vi "RBVASS2mk3.vi"() -> ()   [LabVIEW 2021]
uses:
  <vilib>/myRIO/Instrument Drivers/Onboard IO/AI/AI.lvlib
  <vilib>/myRIO/Common/Instrument Driver Framework/Utilities/typedefs/Analog Scaling Constants.ctl
  <vilib>/myRIO/Common/Instrument Driver Framework/Utilities/typedefs/Analog Scaling Constants List.ctl
  <vilib>/myRIO/Common/Instrument Driver Framework/myRIO v1.0/AI/typedefs/AI Channels Enum.ctl
  <vilib>/myRIO/Common/Instrument Driver Framework/myRIO v1.0/AI/typedefs/AI Channels List.ctl
  <vilib>/myRIO/Common/Instrument Driver Framework/Utilities/typedefs/Generic FPGA Reference.ctl
  <vilib>/myRIO/Common/Instrument Driver Framework/Utilities/typedefs/myRIO v1.0 Reference.ctl
  <vilib>/myRIO/Common/Instrument Driver Framework/Utilities/typedefs/Hardware Version Enum.ctl
  <vilib>/myRIO/Common/Instrument Driver Framework/Utilities/typedefs/myRIO Generic Hardware Reference.ctl
  <vilib>/myRIO/Instrument Drivers/Onboard IO/AI/typedefs/AI Reference.ctl
  <vilib>/myRIO/Instrument Drivers/Onboard IO/AI/vis/myRIO AI Open.xnode
  <vilib>/myRIO/Common/Instrument Driver Framework/myRIO v1.0/AI/vis/myRIO v1.1 Open AI.vi
  <vilib>/userDefined/High Color/nirio_resource_hc.ctl
  <vilib>/vision/driver/NI_Vision_Acquisition_Software.lvlib
  <vilib>/vision/NI_Vision_Development_Module.lvlib
  <vilib>/myRIO/Instrument Drivers/Onboard IO/PWM/PWM.lvlib
  <vilib>/vision/driver/IMAQdx.llb/IMAQdx Camera Control Mode.ctl
  <vilib>/vision/driver/IMAQdx.llb/IMAQdx Acquisition Mode.ctl
  <vilib>/vision/driver/IMAQdx.llb/IMAQdx Buffer Number Mode.ctl
  <vilib>/myRIO/Instrument Drivers/Onboard IO/PWM/typedefs/PWM Configuration.ctl
  <vilib>/myRIO/Common/Instrument Driver Framework/myRIO v1.0/PWM/typedefs/PWM Channels Enum.ctl
  <vilib>/myRIO/Instrument Drivers/Onboard IO/PWM/typedefs/PWM Reference.ctl
  <vilib>/myRIO/Instrument Drivers/Onboard IO/PWM/vis/myRIO PWM Open.xnode
  <vilib>/myRIO/Common/Instrument Driver Framework/myRIO v1.0/PWM/vis/myRIO v1.1 Open PWM.vi
  <vilib>/userDefined/High Color/IMAQdx.ctl
  <vilib>/myRIO/Instrument Drivers/Onboard IO/DIO/DIO.lvlib
  Example VI (1)/t_state.ctl
  <vilib>/myRIO/Common/Instrument Driver Framework/myRIO v1.0/DIO/typedefs/DIO Channels Enum.ctl
  <vilib>/myRIO/Common/Instrument Driver Framework/myRIO v1.0/DIO/typedefs/DIO Channels List.ctl
  <vilib>/myRIO/Instrument Drivers/Onboard IO/DIO/typedefs/DIO Reference.ctl
  <vilib>/myRIO/Common/Instrument Driver Framework/myRIO v1.0/DIO/vis/myRIO v1.1 Open DIO.vi
  <vilib>/myRIO/Instrument Drivers/Onboard IO/DIO/vis/myRIO DIO Open.xnode
  Example VI (1)/t_conn.ctl
panel:
  out "circles":i32
  in  "ROI Descriptor":T1 {"Contours"."Type" items=["No Selection", "Point", "Line", "Rectangle", "Oval", "Polygon", "Freehand Region", "Annulus", "Unused2", "Unused3", "Broken Line", "Freehand Line", "Rotated Rectangle"]}
  out "Image 2":T2(plugin-control)
  in  "error in 2":errorcluster
  in  "Settings":T3={"Objects"=0, "Threshold"=128, "Reject Border"=FALSE, "Fill Holes"=FALSE, "Min Object Size"=FALSE, "Min Size"=3, "Max Object Size"=FALSE, "Max Size"=100, "Show Search Area"=FALSE, "Show Center"=TRUE, "Show Bounding Box"=TRUE} {"Objects" items=["Bright Objects", "Dark Objects"]; "Threshold" min=1 max=999999999 step=1; "Max Size" min=1 max=999999999 step=1; "Min Size" min=1 max=999999999 step=1}
  in  "error in":errorcluster
  in  "stop":bool
  out "object":i32
  out "Colour Value":u32
  out "Color Box":u32(colorbox)
  in  "Knob":dbl(knob) scale=0.0..180.0
  out "error out":errorcluster
  out "Slide":dbl(slide) scale=0.0..10.0
  out "Numeric":i32
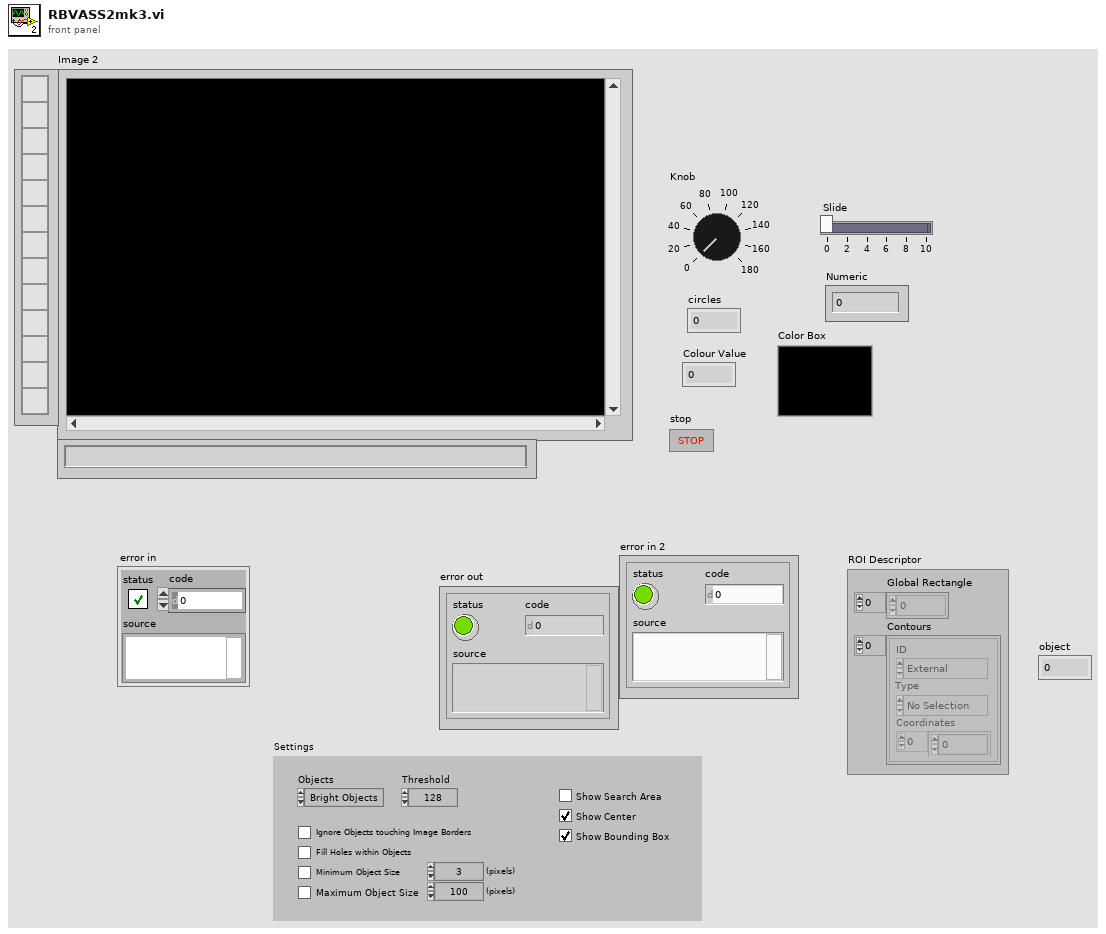
[diagram p1: front panel]
types:
  T1 = cluster{"Global Rectangle":i32[], "Contours":cluster{"ID":enum32{"External", "Internal"}, "Type":u32, "Coordinates":i32[]}[]}
  T2 = typedef "IMAQ Image.ctl" = refnum<image>
  T3 = cluster{"Objects":u16, "Threshold":i32, "Reject Border":bool, "Fill Holes":bool, "Min Object Size":bool, "Min Size":i32, "Max Object Size":bool, "Max Size":i32, "Show Search Area":bool, "Show Center":bool, "Show Bounding Box":bool}
  T4 = typedef "t_conn.ctl" = cluster{"ID":refnum<k5>, "Conn.":bool}
  T5 = typedef "t_state.ctl" = enum16{"Wait for Disconnect", "Stop Listen", "Listen", "Start Listen"}
  T6 = typedef "IMAQdx.ctl" = refnum<k21>
  T7 = typedef "NI_Vision_Acquisition_Software.lvlib/IMAQdx Buffer Number Mode.ctl" = enum32{"Next", "Last", "Buffer Number", "Every", "Last New"}
  T8 = typedef "NI_Vision_Acquisition_Software.lvlib/IMAQdx Acquisition Mode.ctl" = enum32{"One Shot", "Continuous"}
  T9 = typedef "NI_Vision_Acquisition_Software.lvlib/IMAQdx Camera Control Mode.ctl" = enum32{"Controller", "Listener"}
  T10 = typedef "DIO.lvlib/DIO Reference.ctl" = cluster{"myRIO Reference":T11, "DIO Channels List":T15}
  T11 = typedef "myRIO Generic Hardware Reference.ctl" = cluster{"myRIO Model":T12, "myRIO Hardware Reference":T13}
  T12 = typedef "Hardware Version Enum.ctl" = enum16{"Unknown", "myRIO-1900", "myRIO-1950", "roboRIO", "NI ELVIS RIO CM", "ELVIS III"}
  T13 = typedef "myRIO v1.0 Reference.ctl" = cluster{"Generic FPGA Reference":T14, "Allow multiple opens":bool}
  T14 = typedef "Generic FPGA Reference.ctl" = refnum<k20>
  T15 = typedef "DIO Channels List.ctl" = T16[]
  T16 = typedef "DIO Channels Enum.ctl" = enum16{"Not Connected", "C/DIO0", "C/DIO1", "C/DIO2", "C/DIO3", "C/DIO4", "C/DIO5", "C/DIO6", "C/DIO7", "A/DIO0", "A/DIO1", "A/DIO2", "A/DIO3", "A/DIO4", "A/DIO5", "A/DIO6", "A/DIO7", "A/DIO8", "A/DIO9", "A/DIO10", "A/DIO11", "A/DIO12", "A/DIO13", "A/DIO14", "A/DIO15", "A/DIO16", "A/DIO17", "A/DIO18", "A/DIO19", "B/DIO0", "B/DIO1", "B/DIO2", "B/DIO3", "B/DIO4", "B/DIO5", "B/DIO6", "B/DIO7", "B/DIO8", "B/DIO9", "B/DIO10", "B/DIO11", "B/DIO12", "B/DIO13", "B/DIO14", "B/DIO15", "B/DIO16", "B/DIO17", "B/DIO18", "B/DIO19", "LED0", "LED1", "LED2", "LED3", "Button0", "DIO/DIO0", "DIO/DIO1", "DIO/DIO2", "DIO/DIO3", "DIO/DIO4", "DIO/DIO5", "DIO/DIO6", "DIO/DIO7", "DIO/DIO8", "DIO/DIO9", "SPI/CS0", "SPI/CS1", "SPI/CS2", "SPI/CS3", "LED RADIO (Green)", "LED RADIO (Red)", "LED COMM (Green)", "LED COMM (Red)", "LED MODE (Green)", "LED MODE (Red)"}
  T17 = typedef "PWM.lvlib/PWM Reference.ctl" = cluster{"myRIO Reference":T11, "PWM Channels Enum":T18, "PWM Configuration":T19}
  T18 = typedef "PWM Channels Enum.ctl" = enum16{"Not Connected", "C/PWM0", "C/PWM1", "A/PWM0", "A/PWM1", "A/PWM2", "A/PWM3", "A/PWM4", "A/PWM5", "A/PWM6", "A/PWM7", "A/PWM8", "A/PWM9", "A/PWM10", "A/PWM11", "A/PWM12", "A/PWM13", "A/PWM14", "A/PWM15", "A/PWM16", "A/PWM17", "A/PWM18", "A/PWM19", "B/PWM0", "B/PWM1", "B/PWM2", "B/PWM3", "B/PWM4", "B/PWM5", "B/PWM6", "B/PWM7", "B/PWM8", "B/PWM9", "B/PWM10", "B/PWM11", "B/PWM12", "B/PWM13", "B/PWM14", "B/PWM15", "B/PWM16", "B/PWM17", "B/PWM18", "B/PWM19", "PWM/PWM0", "PWM/PWM1", "PWM/PWM2", "PWM/PWM3", "PWM/PWM4", "PWM/PWM5", "PWM/PWM6", "PWM/PWM7", "PWM/PWM8", "PWM/PWM9"}
  T19 = typedef "PWM.lvlib/PWM Configuration.ctl" = cluster{"Frequency":dbl, "Duty Cycle":dbl}
  T20 = typedef "AI.lvlib/AI Reference.ctl" = cluster{"myRIO Reference":T11, "AI Channels List":T21, "AI Scaling Constants List":T23}
  T21 = typedef "AI Channels List.ctl" = T22[]
  T22 = typedef "AI Channels Enum.ctl" = enum16{"Not Connected", "AudioIn/Left", "AudioIn/Right", "C/AI0", "C/AI1", "A/AI0", "A/AI1", "A/AI2", "A/AI3", "A/AI4", "A/AI5", "A/AI6", "A/AI7", "B/AI0", "B/AI1", "B/AI2", "B/AI3", "B/AI4", "B/AI5", "B/AI6", "B/AI7", "AI/AI0", "AI/AI1", "AI/AI2", "AI/AI3", "A/AI0 (DIFF)", "A/AI1 (DIFF)", "A/AI2 (DIFF)", "A/AI3 (DIFF)", "B/AI0 (DIFF)", "B/AI1 (DIFF)", "B/AI2 (DIFF)", "B/AI3 (DIFF)"}
  T23 = typedef "Analog Scaling Constants List.ctl" = T24[]
  T24 = typedef "Analog Scaling Constants.ctl" = cluster{"LSB Weight (Volts)":dbl, "Offset (Volts)":dbl, "Signed?":bool}
  T25 = typedef "Image Type" = u32
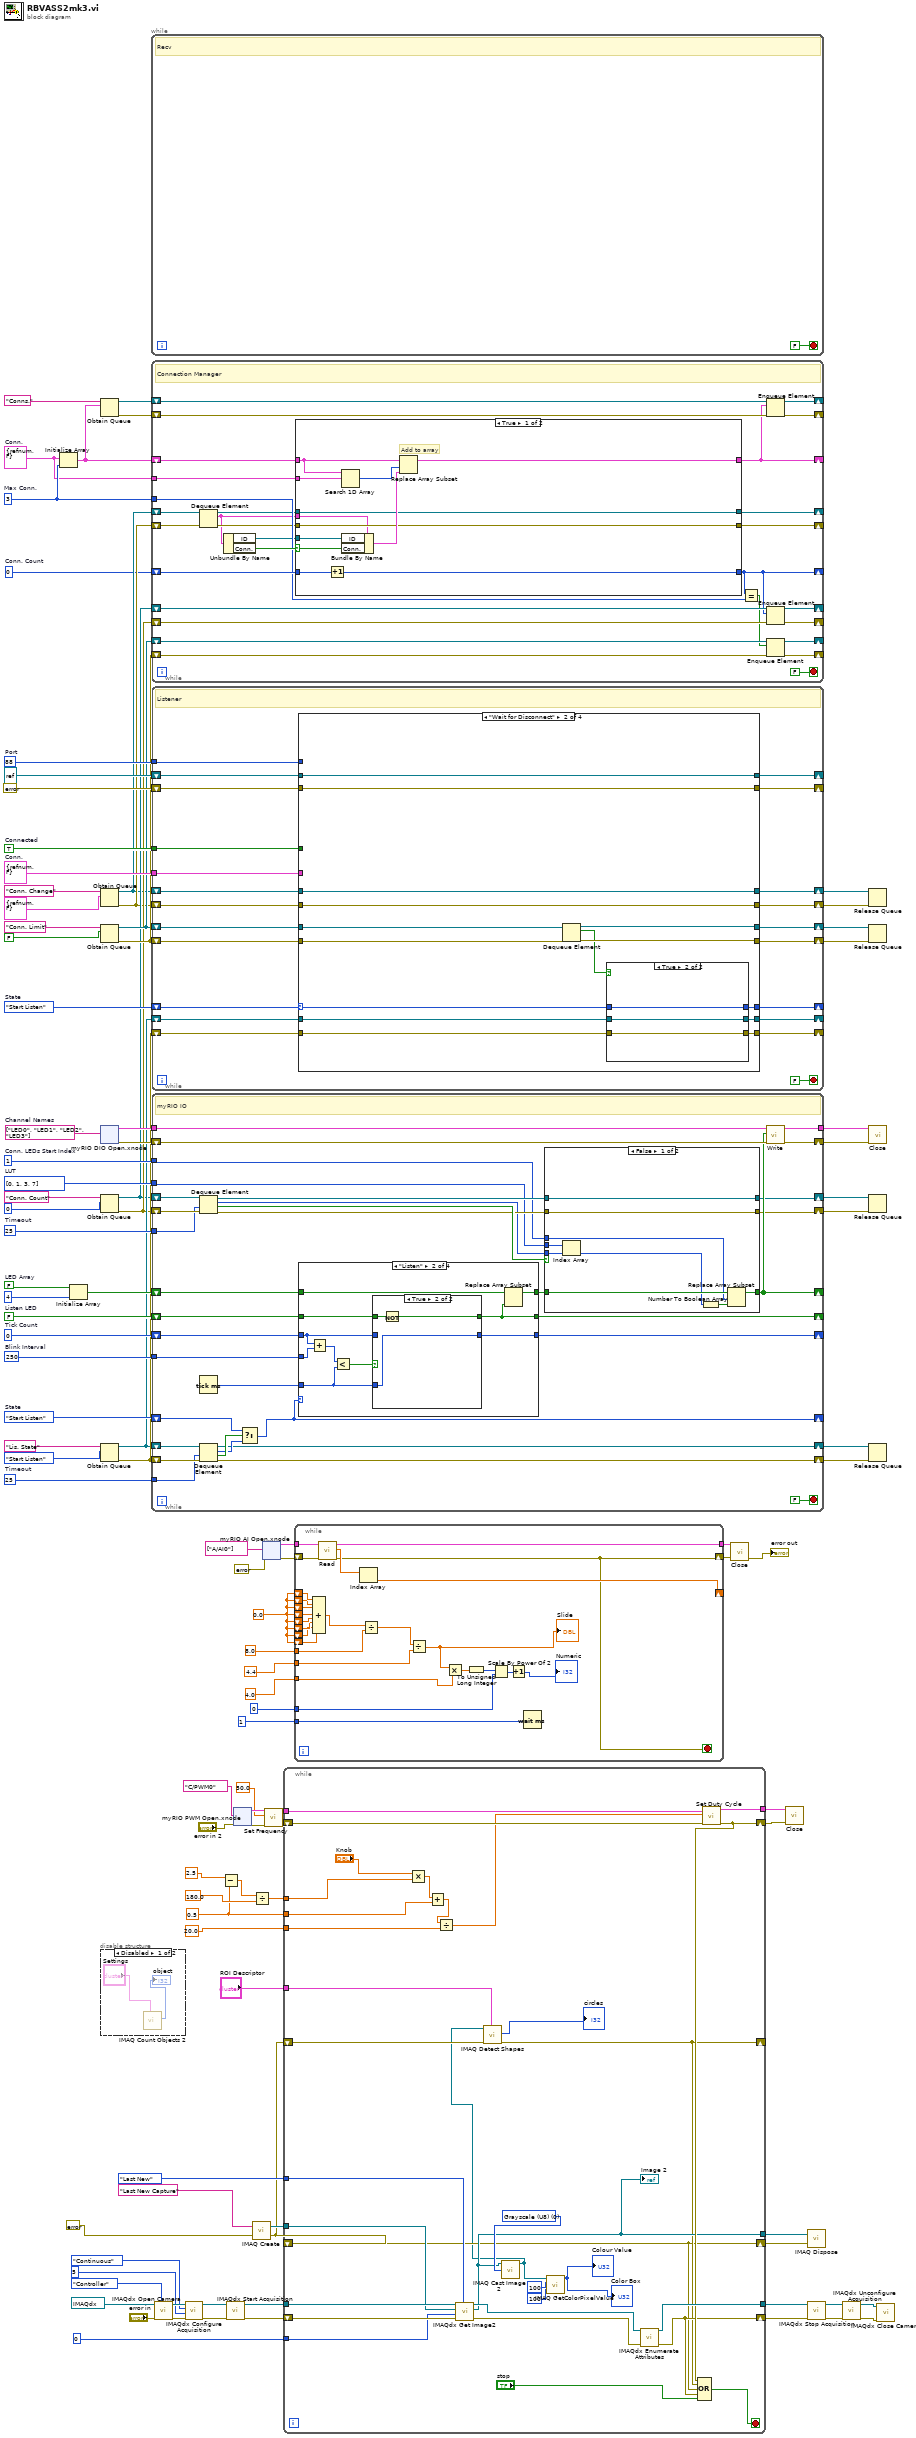
[diagram p0: block diagram]
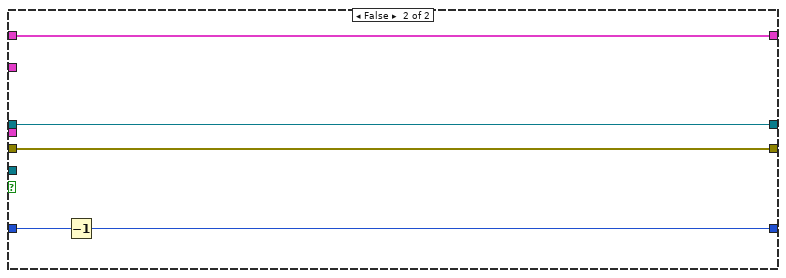
[diagram p2: hidden frame]
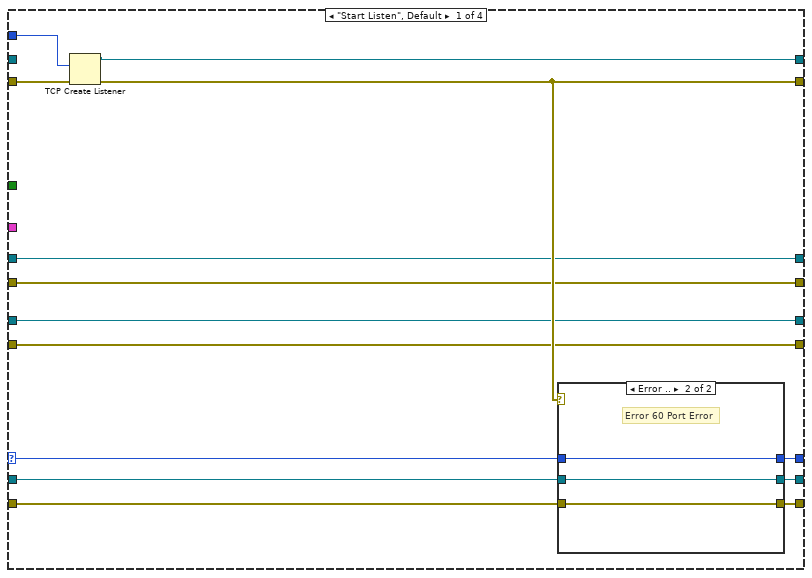
[diagram p3: hidden frame]
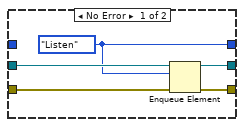
[diagram p4: hidden frame]
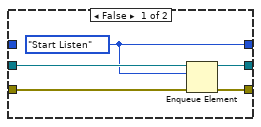
[diagram p5: hidden frame]
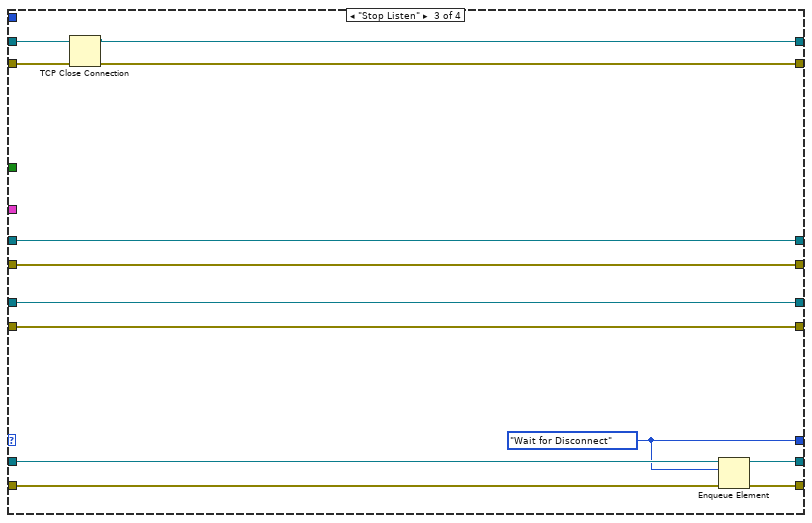
[diagram p6: hidden frame]
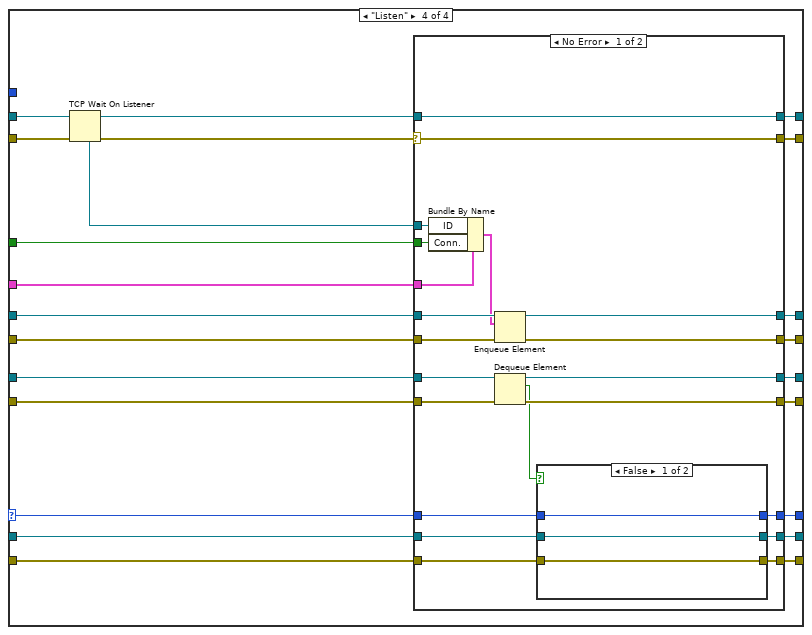
[diagram p7: hidden frame]
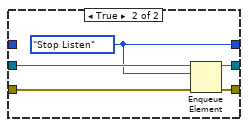
[diagram p8: hidden frame]
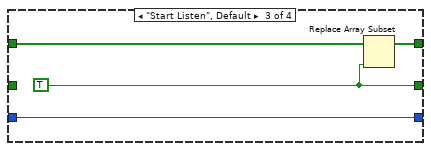
[diagram p13: hidden frame]
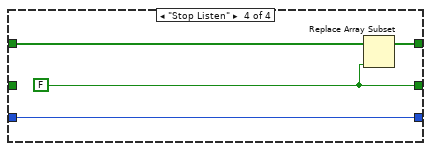
[diagram p14: hidden frame]
diagram:
  w3 = 0  # Conn. Count
  w2 = 3  # Max Conn.
  w1 = T4 {"ID"=refnum, "Conn."=FALSE}  # Conn.
  w18 = TRUE  # Connected
  w24 = u16 88  # Port
  w27 = t_state."Start Listen"  # State
  w19 = T4 {"ID"=refnum, "Conn."=FALSE}  # Conn.
  w32 = 25  # Timeout
  w37 = 25  # Timeout
  w40 = u32 250  # Blink Interval
  w41 = u32 0  # Tick Count
  w42 = t_state."Start Listen"  # State
  w43 = FALSE  # Listen LED
  w44 = i32[] [0, 1, 3, 7]  # LUT
  w45 = 1  # Conn. LEDs Start Index
  w46 = tag[] ["LED0", "LED1", "LED2", "LED3"]  # Channel Names
  w48 = FALSE  # LED Array
  w57 = 0.5
  w101 = 0.0
  n1 = Initialize Array(w1, w2) -> (w4:T4[])
  n2 = Initialize Array(w48, 4 ("dimension size")) -> (w47:bool[])
  n3 = Obtain Queue(name (unnamed)="Conns.", element data type=w4) -> (queue out=w6:refnum<queue>, error out=w7:errorcluster)  [unwired: 3 in, 1 out]
  n4 = Obtain Queue(name (unnamed)="Conn. Change", element data type=T4 {"ID"=refnum, "Conn."=FALSE} ("Conn.")) -> (queue out=w8:refnum<queue>, error out=w9:errorcluster)  [unwired: 3 in, 1 out]
  n5 = Obtain Queue(name (unnamed)="Conn. Limit", element data type=FALSE) -> (queue out=w12:refnum<queue>, error out=w13:errorcluster)  [unwired: 3 in, 1 out]
  n6 = xnode "myRIO DIO Open.xnode"("Channel Names"=w46) -> ("error out"=w53:errorcluster, "DIO Ref Out"=w51:T10)  [unwired: 2 in]
  n7 = Obtain Queue(name (unnamed)="Conn. Count", element data type=0) -> (queue out=w10:refnum<queue>, error out=w11:errorcluster)  [unwired: 3 in, 1 out]
  n8 = Obtain Queue(name (unnamed)="Lis. State", element data type=t_state."Start Listen" ("State")) -> (queue out=w28:refnum<queue>, error out=w29:errorcluster)  [unwired: 3 in, 1 out]
  n9 = disable-structure shown="Disabled" {
    frame Disabled {
      n10 = call "IMAQ Count Objects 2"("Settings"="Settings") -> ("Number of Objects"=→"object":i32)  [unwired: 6 in, 4 out]
    }
    frame Enabled {
    }
  }
  n11 = while {
    stop <- FALSE stop-if-true
    # "Recv"
  }
  n12 = while {
    shift-right: [w135] -> _
    shift-left: w13 -> [w136]
    shift-right: [w133] -> _
    shift-left: w12 -> [w134]
    shift-right: [w131] -> _
    shift-left: w11 -> [w132]
    shift-right: [w129] -> _
    shift-left: w10 -> [w130]
    shift-right: [w113] -> _
    shift-left: w8 -> [w137]
    shift-right: [w115] -> _
    shift-left: w9 -> [w138]
    shift-right: [w125] -> _
    shift-left: w6 -> [w126]
    shift-right: [w127] -> _
    shift-left: w7 -> [w128]
    shift-right: [w111] -> _
    shift-left: w4 -> [w119]
    shift-right: [w122] -> _
    shift-left: w3 -> [w123]
    tunnel: w2 -> [w120]
    tunnel: w1 -> [w118]
    stop <- FALSE stop-if-true
    # "Connection Manager"
    n13 = Dequeue Element(queue=w137, error in (no error)=w138) -> (queue out=w114:refnum<queue>, element=w112:T4, error out=w116:errorcluster)  [unwired: 1 in, 1 out]
    n14 = Unbundle By Name(w112) -> ("ID"=w117:refnum<k5>, "Conn."=w124:bool)
    n15 = case shown="True" w124 {
      selector: w124 -> [w145 _]
      tunnel: w123 -> [w151 w156]
      tunnel: [w150 w155] -> w122
      tunnel: w119 -> [w149 w152]
      tunnel: w118 -> [w146 _]
      tunnel: [w148 w152] -> w111
      tunnel: w117 -> [w144 _]
      tunnel: [w142 w154] -> w115
      tunnel: w116 -> [w142 w154]
      tunnel: w114 -> [w141 w153]
      tunnel: [w141 w153] -> w113
      tunnel: w112 -> [w140 _]
      frame True {
        # "Add to array"
        n16 = Increment(x=w151) -> (x+1=w150:i32)
        n17 = Search 1D Array(1D array=w149, element=w146) -> (index of element=w147:i32)  [unwired: 1 in]
        n18 = Bundle By Name(cluster=w140, "ID"=w144, "Conn."=w145) -> (w143:T4)
        n19 = Replace Array Subset(array=w149, new element=w143, index=w147) -> (w148:T4[])
      }
      frame False {
        n20 = Decrement(x=w156) -> (x-1=w155:i32)
      }
    }
    n21 = Equal?(x=w122, y=w120) -> (x = y?=w121:bool)
    n22 = Enqueue Element(queue=w126, element=w111, error in (no error)=w128) -> (queue out=w125:refnum<queue>, error out=w127:errorcluster)  [unwired: 1 in, 1 out]
    n23 = Enqueue Element(queue=w130, element=w122, error in (no error)=w132) -> (queue out=w129:refnum<queue>, error out=w131:errorcluster)  [unwired: 1 in, 1 out]
    n24 = Enqueue Element(queue=w134, element=w121, error in (no error)=w136) -> (queue out=w133:refnum<queue>, error out=w135:errorcluster)  [unwired: 1 in, 1 out]
  }
  n25 = while {
    shift-right: [w170] -> _
    shift-left: w29 -> [w171]
    shift-right: [w168] -> _
    shift-left: w28 -> [w169]
    shift-right: [w167] -> _
    shift-left: w27 -> [w177]
    shift-right: [w174] -> _
    shift-left: refnum<k5> refnum ("listener ID") -> [w175]
    shift-right: [w173] -> _
    shift-left: errorcluster {"status"=FALSE, "code"=0, "source"=""} ("error constant") -> [w176]
    tunnel: w24 -> [w172]
    shift-right: [w159] -> w14
    shift-left: w8 -> [w160]
    shift-right: [w161] -> w15
    shift-left: w9 -> [w162]
    shift-right: [w163] -> w16
    shift-left: w12 -> [w164]
    shift-right: [w165] -> w17
    shift-left: w13 -> [w166]
    tunnel: w19 -> [w158]
    tunnel: w18 -> [w157]
    stop <- FALSE stop-if-true
    # "Listener"
    n26 = case shown="\"Wait for Disconnect\"" w177 {
      selector: w177 -> [w183 w210 _ w252]
      tunnel: w176 -> [w192 w206 w236 w259]
      tunnel: w175 -> [_ w207 w224 w251]
      tunnel: [w191 w207 w235 w249] -> w174
      tunnel: [w189 w206 w234 w248] -> w173
      tunnel: w172 -> [w190 _ _ _]
      tunnel: w171 -> [w188 w215 w233 w257]
      tunnel: [w187 w214 w232 w256] -> w170
      tunnel: w169 -> [w186 w213 w231 w255]
      tunnel: [w185 w212 w230 w254] -> w168
      tunnel: [w184 w211 w229 w253] -> w167
      tunnel: w166 -> [w182 w205 w228 w247]
      tunnel: [w182 w204 w228 w246] -> w165
      tunnel: w164 -> [w181 w203 w227 w245]
      tunnel: [w181 w202 w227 w244] -> w163
      tunnel: w162 -> [w180 w209 w226 w243]
      tunnel: [w180 w209 w226 w242] -> w161
      tunnel: w160 -> [w179 w208 w225 w241]
      tunnel: [w179 w208 w225 w240] -> w159
      tunnel: w158 -> [_ _ _ w239]
      tunnel: w157 -> [_ _ _ w237]
      frame "Start Listen", Default {
        n27 = TCP Create Listener(8:w192, 10:w190) -> (0:w189:errorcluster, 3:w191:refnum<k5>)  [unwired: 3 in, 1 out]
        n28 = case shown="Error .." w189 {
          tunnel: w188 -> [w197 w198]
          tunnel: [w196 w198] -> w187
          tunnel: w186 -> [w195 w199]
          tunnel: [w194 w199] -> w185
          tunnel: [w193 w200] -> w184
          tunnel: w183 -> [_ w200]
          frame No Error {
            w193 = t_state."Listen" ("State")
            n29 = Enqueue Element(queue=w195, element=w193, error in (no error)=w197) -> (queue out=w194:refnum<queue>, error out=w196:errorcluster)  [unwired: 1 in, 1 out]
          }
          frame Error {
            # "Error 60 Port Error"
          }
        }
      }
      frame "Wait for Disconnect" {
        n30 = Dequeue Element(queue=w203, error in (no error)=w205) -> (queue out=w202:refnum<queue>, element=w201:bool, error out=w204:errorcluster)  [unwired: 1 in, 1 out]
        n31 = case shown="True" w201 {
          tunnel: w215 -> [w220 w221]
          tunnel: [w219 w221] -> w214
          tunnel: w213 -> [w218 w222]
          tunnel: [w217 w222] -> w212
          tunnel: [w216 w223] -> w211
          tunnel: w210 -> [_ w223]
          frame False {
            w216 = t_state."Start Listen" ("State")
            n32 = Enqueue Element(queue=w218, element=w216, error in (no error)=w220) -> (queue out=w217:refnum<queue>, error out=w219:errorcluster)  [unwired: 1 in, 1 out]
          }
          frame True {
          }
        }
      }
      frame "Stop Listen" {
        w229 = t_state."Wait for Disconnect" ("State")
        n33 = TCP Close Connection(connection ID=w224, error in (no error)=w236) -> (connection ID out=w235:refnum<k5>, error out=w234:errorcluster)  [unwired: 1 in]
        n34 = Enqueue Element(queue=w231, element=w229, error in (no error)=w233) -> (queue out=w230:refnum<queue>, error out=w232:errorcluster)  [unwired: 1 in, 1 out]
      }
      frame "Listen" {
        n35 = TCP Wait On Listener(8:w259, 11:w251) -> (0:w258:errorcluster, 3:w250:refnum<k5>, 4:w238:refnum<k5>)  [unwired: 2 in, 2 out]
        n36 = case shown="No Error" w258 {
          selector: w258 -> [w275 w293]
          tunnel: w257 -> [w280 w295]
          tunnel: [w279 w295] -> w256
          tunnel: w255 -> [w278 w296]
          tunnel: [w277 w296] -> w254
          tunnel: [w276 w297] -> w253
          tunnel: w252 -> [w264 w297]
          tunnel: w250 -> [w274 w294]
          tunnel: [w274 w294] -> w249
          tunnel: [w275 w293] -> w248
          tunnel: w247 -> [w273 w292]
          tunnel: [w272 w292] -> w246
          tunnel: w245 -> [w271 w291]
          tunnel: [w270 w291] -> w244
          tunnel: w243 -> [w269 w290]
          tunnel: [w268 w290] -> w242
          tunnel: w241 -> [w266 w289]
          tunnel: [w267 w289] -> w240
          tunnel: w239 -> [w263 _]
          tunnel: w238 -> [w262 _]
          tunnel: w237 -> [w261 _]
          frame No Error {
            n37 = Bundle By Name(cluster=w263, "ID"=w262, "Conn."=w261) -> (w260:T4)
            n38 = Enqueue Element(queue=w266, element=w260, error in (no error)=w269) -> (queue out=w267:refnum<queue>, error out=w268:errorcluster)  [unwired: 1 in, 1 out]
            n39 = Dequeue Element(queue=w271, error in (no error)=w273) -> (queue out=w270:refnum<queue>, element=w265:bool, error out=w272:errorcluster)  [unwired: 1 in, 1 out]
            n40 = case shown="False" w265 {
              tunnel: w280 -> [w283 w288]
              tunnel: [w283 w287] -> w279
              tunnel: w278 -> [w282 w286]
              tunnel: [w282 w285] -> w277
              tunnel: [w281 w284] -> w276
              tunnel: w264 -> [w281 _]
              frame False {
              }
              frame True {
                w284 = t_state."Stop Listen" ("State")
                n41 = Enqueue Element(queue=w286, element=w284, error in (no error)=w288) -> (queue out=w285:refnum<queue>, error out=w287:errorcluster)  [unwired: 1 in, 1 out]
              }
            }
          }
          frame Error {
          }
        }
      }
    }
  }
  n42 = while {
    shift-right: [w329] -> w52
    shift-left: w53 -> [w330]
    tunnel: w51 -> [w328]
    tunnel: [w327] -> w50
    shift-right: [w318] -> _
    shift-left: w47 -> [w326]
    tunnel: w45 -> [w307]
    tunnel: w44 -> [w308]
    shift-right: [w324] -> _
    shift-left: w43 -> [w325]
    shift-right: [w300] -> _
    shift-left: w42 -> [w301]
    shift-right: [w321] -> _
    shift-left: w41 -> [w322]
    tunnel: w40 -> [w320]
    shift-right: [w310] -> w35
    shift-left: w10 -> [w316]
    shift-right: [w312] -> w36
    shift-left: w11 -> [w317]
    tunnel: w37 -> [w315]
    shift-right: [w298] -> w30
    shift-left: w28 -> [w306]
    shift-right: [w299] -> w31
    shift-left: w29 -> [w305]
    tunnel: w32 -> [w304]
    stop <- FALSE stop-if-true
    # "myRIO IO"
    n43 = Dequeue Element(queue=w316, timeout in ms (-1)=w315, error in (no error)=w317) -> (queue out=w311:refnum<queue>, element=w309:i32, timed out?=w314:bool, error out=w313:errorcluster)
    n44 = Tick Count (ms)() -> (millisecond timer value=w323:u32)
    n45 = Dequeue Element(queue=w306, timeout in ms (-1)=w304, error in (no error)=w305) -> (queue out=w298:refnum<queue>, element=w302:T5, timed out?=w303:bool, error out=w299:errorcluster)
    n46 = Select(t=w301, s=w303, f=w302) -> (s? t:f=w300:T5)
    n47 = case shown="\"Listen\"" w300 {
      tunnel: w326 -> [w344 w356 w365 w369]
      tunnel: [w344 w355 w364 w368] -> w319
      tunnel: w325 -> [w345 w349 _ _]
      tunnel: [w345 w347 w363 w367] -> w324
      tunnel: w323 -> [_ w351 _ _]
      tunnel: w322 -> [w346 w348 w362 w366]
      tunnel: [w346 w350 w362 w366] -> w321
      tunnel: w320 -> [_ w354 _ _]
      frame "Wait for Disconnect" {
      }
      frame "Listen" {
        n48 = Add(x=w348, y=w354) -> (x+y=w353:u32)
        n49 = Less?(x=w353, y=w351) -> (x < y?=w352:bool)
        n50 = case shown="True" w352 {
          tunnel: w351 -> [_ w361]
          tunnel: [w358 w361] -> w350
          tunnel: w349 -> [w357 w360]
          tunnel: [w357 w359] -> w347
          tunnel: w348 -> [w358 _]
          frame False {
          }
          frame True {
            n51 = Not(x=w360) -> (.not. x?=w359:bool)
          }
        }
        n52 = Replace Array Subset(array=w356, new element=w347) -> (w355:bool[])  [unwired: 1 in]
      }
      frame "Start Listen", Default {
        w363 = TRUE
        n53 = Replace Array Subset(array=w365, new element=w363) -> (w364:bool[])  [unwired: 1 in]
      }
      frame "Stop Listen" {
        w367 = FALSE
        n54 = Replace Array Subset(array=w369, new element=w367) -> (w368:bool[])  [unwired: 1 in]
      }
    }
    n55 = case shown="False" w314 {
      tunnel: w319 -> [w336 w343]
      tunnel: [w335 w343] -> w318
      tunnel: w313 -> [w338 w342]
      tunnel: [w338 w342] -> w312
      tunnel: w311 -> [w337 w341]
      tunnel: [w337 w341] -> w310
      tunnel: w309 -> [w340 _]
      tunnel: w308 -> [w339 _]
      tunnel: w307 -> [w334 _]
      frame False {
        n56 = Index Array(array=w339, index=w340) -> (element=w333:i32)
        n57 = Number To Boolean Array(number=w333) -> (Boolean array=w332:bool[])
        n58 = Replace Array Subset(array=w336, new element=w332, index=w334) -> (w335:bool[])
      }
      frame True {
      }
    }
    n59 = call <vilib>:"Write.vi"("error in (no error)"=w330, "Values"=w318, "DIO Ref In"=w328) -> ("error out"=w329:errorcluster, "DIO Ref Out"=w327:T10)  [unwired: 6 in]
  }
  n60 = call <vilib>:"IMAQdx Open Camera.vi"("Camera Control Mode"=IMAQdx_Camera_Control_Mode."Controller", "error in"="error in", "Session In"=T6 "cam0") -> ("error out"=w87:errorcluster, "Session Out"=w88:T6)  [unwired: 7 in]
  n61 = call <vilib>:"IMAQdx Configure Acquisition.vi"("error in"=w87, "Number of Buffers"=u32 5, "Continuous?"=IMAQdx_Acquisition_Mode."Continuous", "Session In"=w88) -> ("error out"=w94:errorcluster, "Session Out"=w93:T6)  [unwired: 6 in]
  n62 = Subtract(x=2.5, y=w57) -> (x-y=w62:dbl)
  n63 = call <vilib>:"IMAQdx Start Acquisition.vi"("error in"=w94, "Session In"=w93) -> ("error out"=w81:errorcluster, "Session Out"=w82:T6)  [unwired: 8 in]
  n64 = xnode "myRIO PWM Open.xnode"("error in (no error)"="error in 2", "Channel Name"=tag "C/PWM0") -> ("error out"=w70:errorcluster, "PWM Ref Out"=w69:T17)  [unwired: 1 in]
  n65 = call "IMAQ Create"("Image Name"="Last New Capture", "error in (no error)"=errorcluster {"status"=FALSE, "code"=0, "source"=""} ("error in")) -> ("New Image"=w78:T2, "error out"=w54:errorcluster)  [unwired: 3 in]
  n66 = Divide(x=w62, y=180.0) -> (x/y=w58:dbl)
  n67 = xnode "myRIO AI Open.xnode"("error in (no error)"=errorcluster {"status"=FALSE, "code"=0, "source"=""}, "Channel Names"=tag[] ["A/AI0"]) -> ("error out"=w106:errorcluster, "AI Ref Out"=w107:T20)  [unwired: 1 in]
  n68 = call <vilib>:"Set Frequency.vi"("error in (no error)"=w70, "Frequency [Hz]"=50.0, "PWM Ref In"=w69) -> ("error out"=w66:errorcluster, "PWM Ref Out"=w64:T17)  [unwired: 6 in]
  n69 = while {
    tunnel: w82 -> [w402]
    shift-right: [w373] -> w76
    shift-left: w81 -> [w401]
    tunnel: w78 -> [w400]
    shift-right: [w371] -> w77
    shift-left: w54 -> [w371]
    tunnel: [w375] -> w75
    tunnel: [w399] -> w74
    tunnel: u32 0 ("Buffer Number In") -> [w397]
    shift-right: [w372] -> _
    shift-left: w54 -> [w378]
    tunnel: IMAQdx_Buffer_Number_Mode."Last New" ("Buffer Number Mode (Next)") -> [w396]
    shift-right: [w386] -> w65
    shift-left: w66 -> [w389]
    tunnel: w64 -> [w388]
    tunnel: [w387] -> w63
    tunnel: w57 -> [w382]
    tunnel: 20.0 -> [w381]
    tunnel: w58 -> [w380]
    tunnel: "ROI Descriptor" -> [w377]
    stop <- w395 stop-if-true
    w390 = T25 0 items=["Grayscale (U8)", "Grayscale (I16)", "Grayscale (SGL)", "Complex (CSG)", "RGB (U32)", "HSL (U32)", "RGB (U64)", "Grayscale (U16)"] ("Image Type")
    n70 = Multiply(x="Knob", y=w380) -> (x*y=w384:dbl)
    n71 = Add(x=w384, y=w382) -> (x+y=w383:dbl)
    n72 = Divide(x=w383, y=w381) -> (x/y=w379:dbl)
    n73 = call <vilib>:"IMAQdx Get Image2.vi"("Buffer Number Mode (Next)"=w396, "error in"=w401, "Buffer Number In"=w397, "Image In"=w400, "Session In"=w402) -> ("error out"=w398:errorcluster, "Image Out"=w375:T2, "Session Out"=w391:T6)  [unwired: 3 in, 1 out]
    "Image 2" <- w375
    n74 = call "IMAQ Cast Image 2"("Image Src"=w375, "Image Type"=w390) -> ("Image Dst Out"=w370:T2)  [unwired: 12 in, 1 out]
    n75 = call-poly "IMAQ Detect Shapes"("ROI Descriptor"=w377, "error in (no error)"=w378, "Image"=w370) -> ("error out"=w372:errorcluster, "Number of Matches Returned"=→"circles":i32)  [unwired: 6 in, 1 out]
    n76 = call "IMAQ GetColorPixelValue"("Y Coordinate"=100, "X Coordinate"=100, "Image"=w370) -> ("Pixel Value (U32)"=→"Colour Value" →"Color Box":u32)  [unwired: 1 in, 2 out]
    n77 = call <vilib>:"IMAQdx Enumerate Attributes.vi"("error in"=w398, "Session In"=w391) -> ("error out"=w373:errorcluster, "Session Out"=w399:T6)  [unwired: 7 in, 1 out]
    n78 = call <vilib>:"Set Duty Cycle.vi"("error in (no error)"=w389, "Duty Cycle"=w379, "PWM Ref In"=w388) -> ("error out"=w386:errorcluster, "PWM Ref Out"=w387:T17)  [unwired: 6 in]
    n79 = Compound Arithmetic op=OR(w386, w372, w371, w373, "stop") -> (w395:bool)
  }
  n80 = while {
    tunnel: w107 -> [w428]
    shift-right: [w412] -> w105
    shift-left: w106 -> [w427]
    tunnel: [w426] -> w104
    shift-right: [w424] -> _
    shift-left: w101 -> [w423]
    shift-left: w101 -> [w422]
    shift-left: w101 -> [w421]
    shift-left: w101 -> [w420]
    shift-left: w101 -> [w419]
    shift-left: w101 -> [w418]
    shift-left: w101 -> [w417]
    shift-left: w101 -> [w416]
    tunnel: 8.0 -> [w414]
    tunnel: u32 1 -> [w413]
    tunnel: 4.4 -> [w410]
    tunnel: 4.0 -> [w408]
    tunnel: 0 -> [w405]
    stop <- w412 stop-if-true
    n81 = Compound Arithmetic op=ADD(w423, w422, w421, w420, w419, w418, w417, w416) -> (w415:dbl)
    n82 = call <vilib>:"Read.vi"("error in (no error)"=w427, "AI Ref In"=w428) -> ("error out"=w412:errorcluster, "Values"=w425:dbl[], "AI Ref Out"=w426:T20)  [unwired: 7 in]
    n83 = Index Array(array=w425) -> (element=w424:dbl)  [unwired: 1 in]
    n84 = Divide(x=w415, y=w414) -> (x/y=w411:dbl)
    n85 = Divide(x=w411, y=w410) -> (x/y=w409:dbl)
    "Slide" <- w409
    n86 = Multiply(x=w409, y=w408) -> (x*y=w407:dbl)
    n87 = To Unsigned Long Integer(number=w407) -> (unsigned 32bit integer=w406:u32)
    n88 = Scale By Power Of 2(n=w406, x=w405) -> (x*2^n=w404:i32)
    n89 = Increment(x=w404) -> (x+1=→"Numeric":i32)
    n90 = Wait (ms)(milliseconds to wait=w413) -> ()  [unwired: 1 out]
  }
  n91 = call <vilib>:"Close.vi"("error in (no error)"=w105, "AI Ref In"=w104) -> ("error out"=→"error out":errorcluster)  [unwired: 9 in]
  n92 = call <vilib>:"Close.vi"("error in (no error)"=w65, "PWM Ref In"=w63) -> ()  [unwired: 9 in, 1 out]
  n93 = call "IMAQ Dispose"("Image"=w75, "error in (no error)"=w77) -> ()  [unwired: 4 in, 1 out]
  n94 = call <vilib>:"IMAQdx Stop Acquisition.vi"("error in"=w76, "Session In"=w74) -> ("error out"=w90:errorcluster, "Session Out"=w91:T6)  [unwired: 8 in]
  n95 = call <vilib>:"IMAQdx Unconfigure Acquisition.vi"("error in"=w90, "Session In"=w91) -> ("error out"=w89:errorcluster, "Session Out"=w92:T6)  [unwired: 8 in]
  n96 = Release Queue(queue=w14, error in (no error)=w15) -> ()  [unwired: 1 in, 3 out]
  n97 = Release Queue(queue=w16, error in (no error)=w17) -> ()  [unwired: 1 in, 3 out]
  n98 = call <vilib>:"Close.vi"("error in (no error)"=w52, "DIO Ref In"=w50) -> ()  [unwired: 9 in, 1 out]
  n99 = Release Queue(queue=w35, error in (no error)=w36) -> ()  [unwired: 1 in, 3 out]
  n100 = Release Queue(queue=w30, error in (no error)=w31) -> ()  [unwired: 1 in, 3 out]
  n101 = call <vilib>:"IMAQdx Close Camera.vi"("error in"=w89, "Session In"=w92) -> ()  [unwired: 9 in, 1 out]
